vi "Get Module Information.vi"(8 "error in":errorcluster, 11 "Module in":refnum<class "Module.lvclass">) -> (0 "error out":errorcluster, 2 "Module Information":T1 {"Module Code" format="%.0x"}, 3 "Module out":refnum<class "Module.lvclass">)   [LabVIEW 2016, in "SMI.lvlib" / "Module.lvclass"]
uses:
  Module.lvclass
  Controls/ModuleInformation.ctl
  C:/GitHub/SystemManagementAndInformation/source/classes/Device/Device.lvclass
  Device/Device.lvclass/Device.ctl
  Device/read vendor name.vi
  Device/read product name.vi
  Device/read product ID.vi
  Device/read serial number.vi
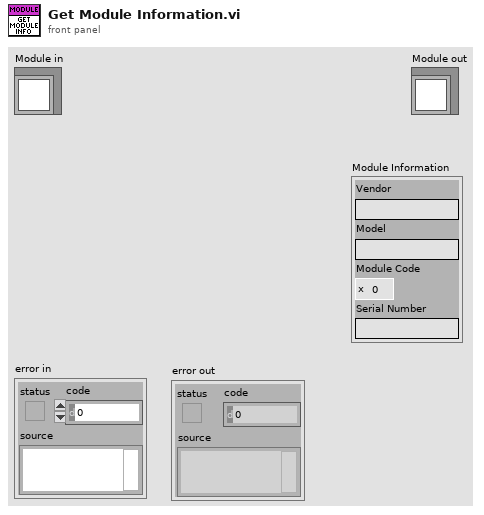
[diagram p1: front panel]
types:
  T1 = typedef "SMI.lvlib/Module.lvclass/ModuleInformation.ctl" = cluster{"Vendor":string, "Model":string, "Module Code":u16, "Serial Number":string}
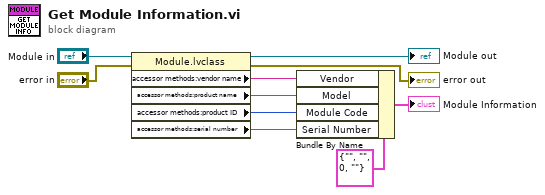
[diagram p0: block diagram]
diagram:
  n1 = property class="Module.lvclass"(reference="Module in", error in="error in") -> (reference out=→"Module out":refnum<class "Module.lvclass">, error out=→"error out":errorcluster, "accessor methods:vendor name"=w6:string, "accessor methods:product name"=w5:string, "accessor methods:product ID"=w1:u16, "accessor methods:serial number"=w4:string)
  n2 = Bundle By Name(cluster=T1 {"Vendor"="", "Model"="", "Module Code"=0, "Serial Number"=""} ("Module Information"), "Vendor"=w6, "Model"=w5, "Module Code"=w1, "Serial Number"=w4) -> (→"Module Information":T1)
